vi "Magnetic Sweep 1.3.vi"() -> ()   [LabVIEW 2011]
uses:
  <vilib>/Math Plots/3D Math Plots/3D Contour/3D Contour XCtrl/3D Contour.xctl
  <vilib>/Math Plots/3D Math Plots/3D Contour/3D Contour Datatype/Public/Plot Helper (Vector).vi
  <vilib>/Math Plots/3D Math Plots/3D Contour/3D Contour Datatype/3D Contour Datatype.lvclass
panel:
  in  "Set parameter":bool
  out "status":string
  out "PID command":string
  out "setpoint command":string
  out "setpoint":dbl
  out "3D Contour \n(Ramp down)":refnum<class "3D Plot Datatype.lvclass">[](xcontrol)
  out "3D Contour\n(Ramp up)":refnum<class "3D Plot Datatype.lvclass">[](xcontrol)
  in  "stop":bool
  out "error out 3":errorcluster
  out "error out 2":errorcluster
  in  "Contour plot (ramp down)":path
  in  "Raw data (ramp down)":path
  out "Elapsed Time (s)":dbl
  out "Numeric":i32
  in  "error out":errorcluster
  out "Initial Temperature":string
  out "Zero field reached":bool
  out "Target field reached":bool
  in  "Upper limite":dbl
  in  "Temperature\nramping step":dbl
  in  "Heater range":i16(ring) items=["High", "Medium", "Low"]
  in  "D gain":dbl
  in  "I gain":dbl
  in  "P gain":dbl
  in  "Contour plot (ramp up)":path
  out "Time elapsed":string
  in  "Timer":bool caption="Reset"
  in  "date format":enum16{"short", "long", "abbreviated"}(ring)
  in  "Save":bool
  in  "Raw data (ramp  up)":path
  out "Temperature vs Time":cluster{dbl[], dbl[]}(graph)
  out "current time":timestamp
  out "Magnetic\nField":cluster{dbl[], dbl[]}(graph)
  out "Current Resistance":string
  out "Current Temperature":string
  out "Current Field":string
  out "Status":string
  in  "Field Sweep":bool
  in  "Magnetic field\nRamp rate":dbl
  in  "Traget Field":dbl
  out "Init Response":string
  in  "error in (no error)":errorcluster
  in  "IP Address":string
  in  "Ramp":bool
  in  "Update":bool
  in  "Ramp to Zero":bool
  in  "P Switch":bool
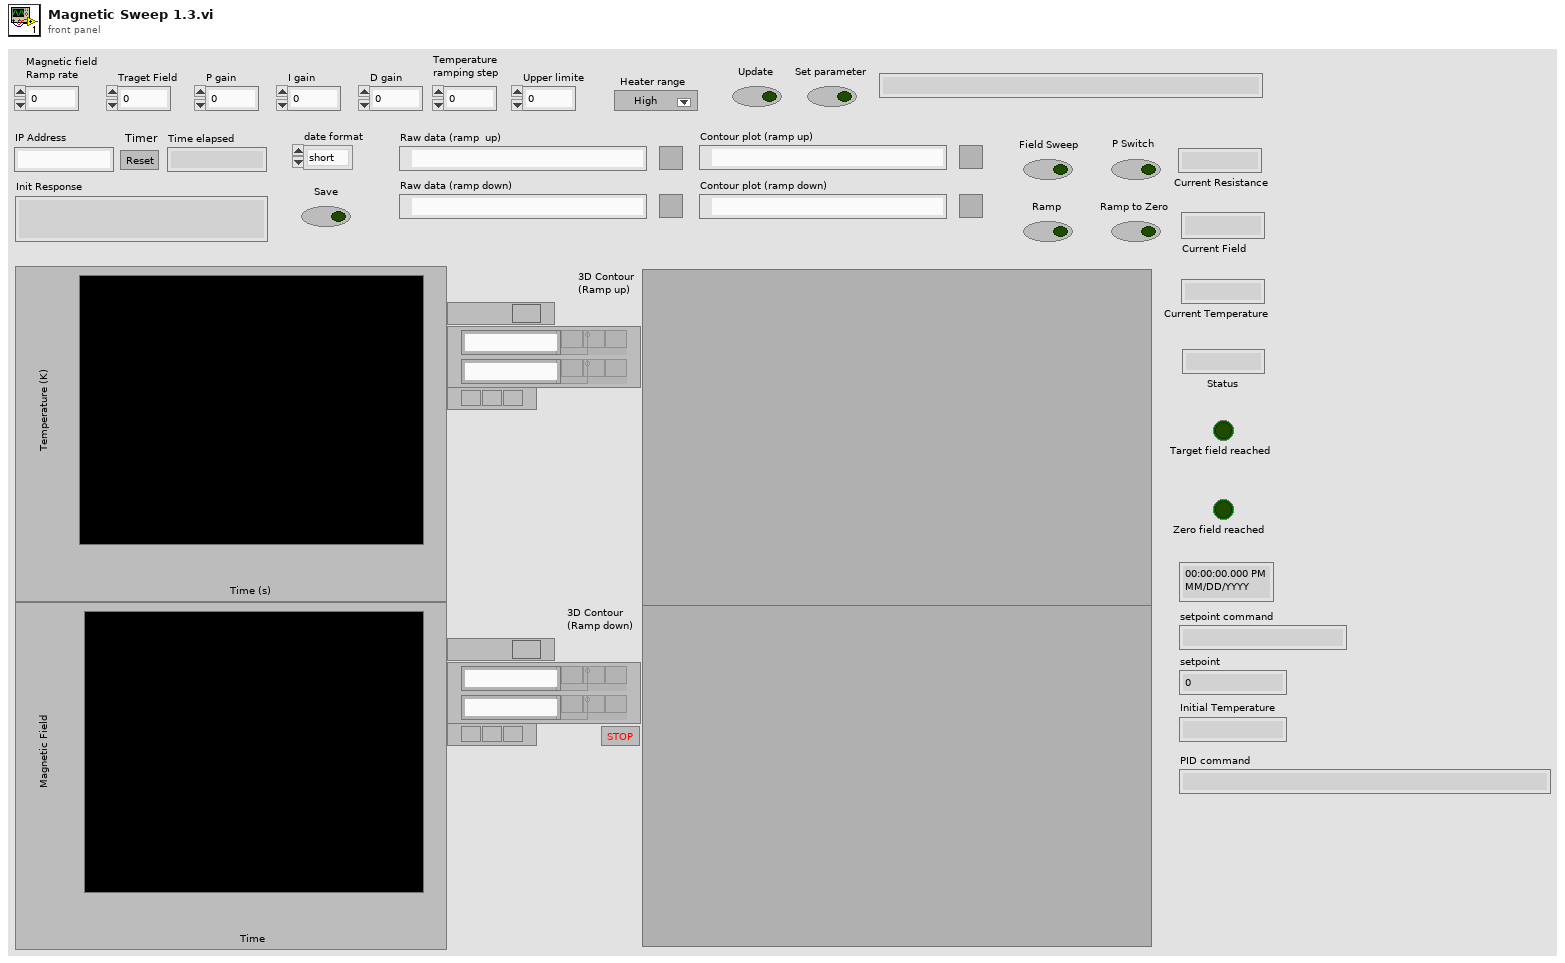
[diagram p1: front panel]
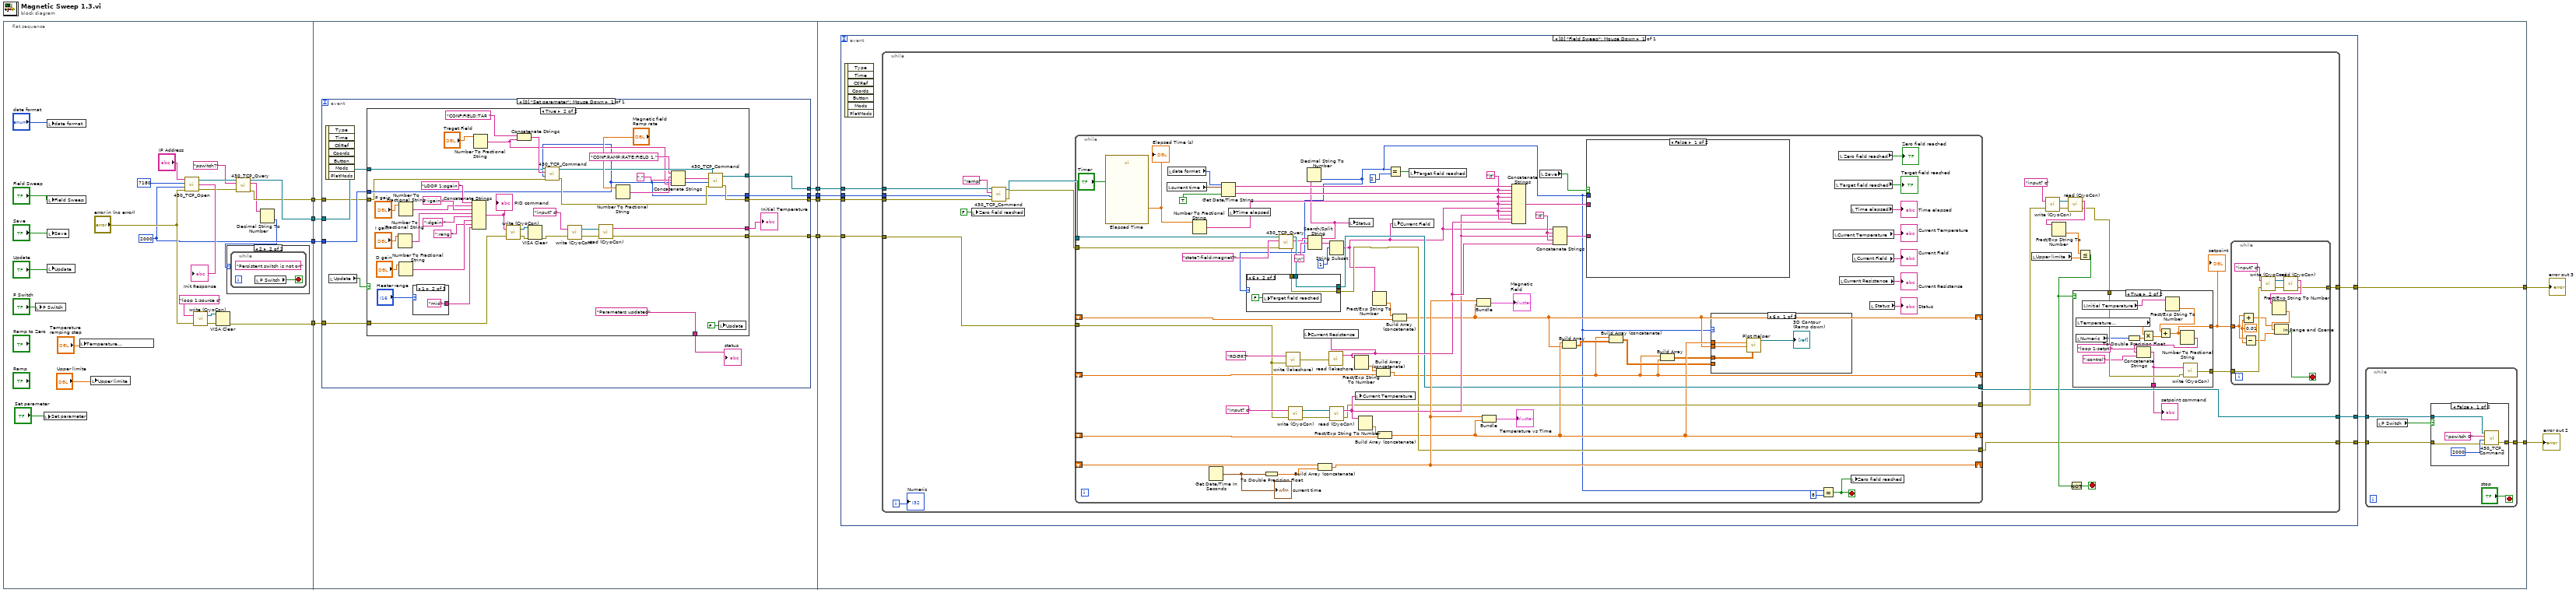
[diagram p0: block diagram]
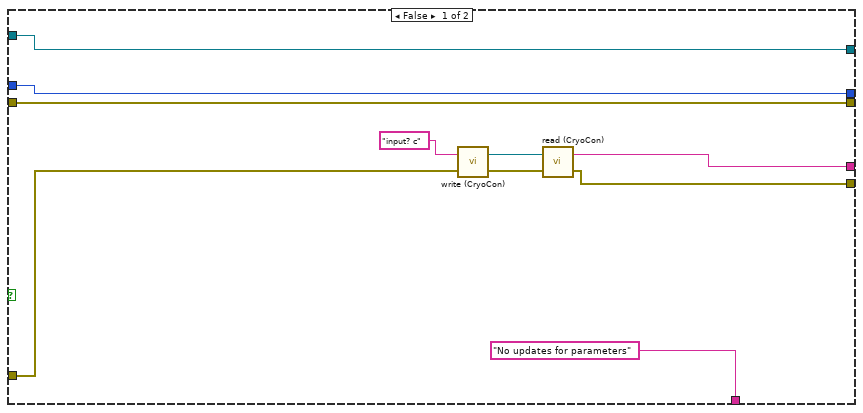
[diagram p3: hidden frame]
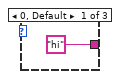
[diagram p4: hidden frame]
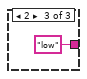
[diagram p5: hidden frame]
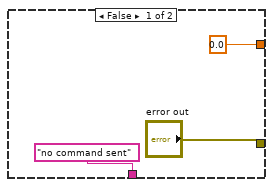
[diagram p7: hidden frame]
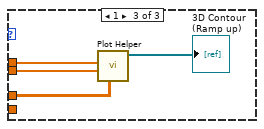
[diagram p9: hidden frame]
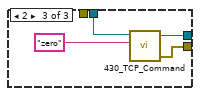
[diagram p11: hidden frame]
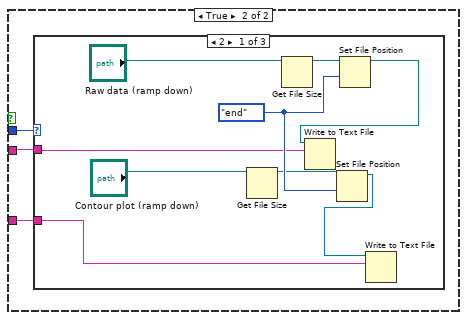
[diagram p12: hidden frame]
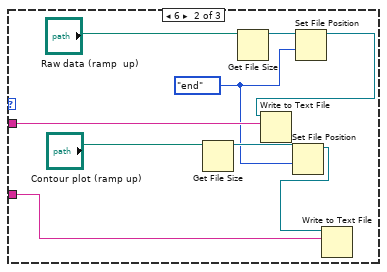
[diagram p13: hidden frame]
diagram:
  n1 = flat-sequence {
    tunnel: [w20] -> w10
    tunnel: [w22] -> w9
    tunnel: [w11] -> w8
    tunnel: [w18] -> w1
    tunnel: w10 -> [w43]
    tunnel: w9 -> [w42]
    tunnel: w8 -> [w41]
    tunnel: [w40] -> w7
    tunnel: [w39] -> w4
    tunnel: [w38] -> w3
    tunnel: [w37] -> w2
    tunnel: w1 -> [w36]
    tunnel: w7 -> [w115]
    tunnel: [w114] -> w6
    tunnel: [w112] -> w5
    tunnel: w4 -> [w110]
    tunnel: w3 -> [w109]
    tunnel: w2 -> [w108]
    frame #0 {
      w22 = 2000 ("Timeout")
      n2 = local write "P Switch"("P Switch") -> ()
      n3 = local write "Set parameter"("Set parameter") -> ()
      n4 = local write "date format"("date format") -> ()
      n5 = local write "Field Sweep"("Field Sweep") -> ()
      n6 = local write "Save"("Save") -> ()
      n7 = local write "Update"("Update") -> ()
      n8 = local write "Temperature\nramping step"("Temperature\nramping step") -> ()
      n9 = local write "Upper limite"("Upper limite") -> ()
      n10 = call "430_TCP_Open.vi"("IP Address"="IP Address", "TCP Port"=7180, "timeout ms (2000)"=w22, "error in (no error)"="error in (no error)") -> ("connection ID"=w21:refnum<k5>, "Init Response"=→"Init Response":string, "error out"=w19:errorcluster)  [unwired: 2 in]
      n11 = call "write (CryoCon).vi"("error in (no error)"="error in (no error)", "write buffer"="loop 1:source c") -> ("error out"=w13:errorcluster, "VISA resource name out"=w12:refnum<visa-resource-name>)
      n12 = VISA Clear(VISA resource name=w12, error in (no error)=w13) -> (error out=w11:errorcluster)  [unwired: 1 out]
      n13 = call "430_TCP_Query.vi"("error in (no error)"=w19, "Command"="pswitch?", "connection ID"=w21) -> ("error out"=w18:errorcluster, "Response"=w16:string, "connection ID out"=w20:refnum<k5>)  [unwired: 4 in, 2 out]
      n14 = Decimal String To Number(string=w16) -> (number=w15:i32)  [unwired: 2 in, 1 out]
      n15 = case shown="2" w15 {
        frame 1, Default {
        }
        frame 2 {
          n16 = while {
            stop <- w35 stop-if-true
            (unwired) "Persistent switch is not on"
            n17 = local read "P Switch"() -> (w35:bool)
          }
        }
      }
    }
    frame #1 {
      n18 = event shown="[0] \"Set parameter\": Mouse Down" {
        selector: _ -> [_]
        dyn-events: _ -> [_]
        timeout: _ -> [_]
        tunnel: w43 -> [w54]
        tunnel: w42 -> [w53]
        tunnel: w41 -> [w52]
        tunnel: [w51] -> w40
        tunnel: [w50] -> w39
        tunnel: [w49] -> w38
        tunnel: [w48] -> w37
        tunnel: w36 -> [w45]
        event "Set parameter": Mouse Down {
          n19 = event-data() -> ()  [unwired: 1 in, 7 out]
          n20 = local read "Update"() -> (w44:bool)
          n21 = case shown="True" w44 {
            tunnel: w54 -> [w62 w102]
            tunnel: w53 -> [w63 w72]
            tunnel: w52 -> [w56 w81]
            tunnel: [w61 w76] -> w51
            tunnel: ["No updates for parameters" ("String") "Parameters updated" ("String")] -> w47
            tunnel: [w55 w74] -> w50
            tunnel: [w62 w73] -> w49
            tunnel: [w63 w72] -> w48
            tunnel: [w58 w71] -> w46
            tunnel: w45 -> [w55 w68]
            frame False {
              n22 = call "write (CryoCon).vi"("error in (no error)"=w56, "write buffer"="input? c") -> ("error out"=w59:errorcluster, "VISA resource name out"=w57:refnum<visa-resource-name>)
              n23 = call "read (CryoCon).vi"("error in (no error)"=w59, "VISA resource name"=w57) -> ("error out"=w61:errorcluster, "read buffer"=w58:string)
            }
            frame True {
              n24 = Number To Fractional String(number="I gain") -> (F-format string=w85:string)  [unwired: 3 in]
              n25 = Number To Fractional String(number="D gain") -> (F-format string=w83:string)  [unwired: 3 in]
              n26 = Number To Fractional String(number="P gain") -> (F-format string=w86:string)  [unwired: 3 in]
              n27 = case shown="1" "Heater range" {
                tunnel: ["hi" "mid" "low"] -> w78
                frame 0, Default {
                }
                frame 1 {
                }
                frame 2 {
                }
              }
              n28 = Concatenate Strings("LOOP 1:pgain " ("write buffer"), w86, ";igain " ("string"), w85, ";dgain " ("string"), w83, ";rang " ("string"), w78) -> (w82:string)
              "PID command" <- w82
              n29 = Number To Fractional String(number="Traget Field") -> (F-format string=w92:string)  [unwired: 3 in]
              n30 = call "write (CryoCon).vi"("error in (no error)"=w81, "write buffer"=w82) -> ("error out"=w67:errorcluster, "VISA resource name out"=w66:refnum<visa-resource-name>)
              n31 = Concatenate Strings("CONF:FIELD:TAR ", w92) -> (w103:string)
              n32 = VISA Clear(VISA resource name=w66, error in (no error)=w67) -> (error out=w65:errorcluster)  [unwired: 1 out]
              n33 = call "430_TCP_Command.vi"("error in (no error)"=w68, "Timeout"=w72, "Command"=w103, "connection ID"=w102) -> ("error out"=w101:errorcluster, "connection ID out"=w97:refnum<k5>)  [unwired: 1 out]
              n34 = call "write (CryoCon).vi"("error in (no error)"=w65, "write buffer"="input? c") -> ("error out"=w77:errorcluster, "VISA resource name out"=w69:refnum<visa-resource-name>)
              n35 = call "read (CryoCon).vi"("error in (no error)"=w77, "VISA resource name"=w69) -> ("error out"=w76:errorcluster, "read buffer"=w71:string)
              n36 = Number To Fractional String(number="Magnetic field\nRamp rate") -> (F-format string=w95:string)  [unwired: 3 in]
              n37 = Concatenate Strings("CONF:RAMP:RATE:FIELD 1," ("string"), w95, "," ("string"), w92) -> (w98:string)
              n38 = call "430_TCP_Command.vi"("error in (no error)"=w101, "Timeout"=w72, "Command"=w98, "connection ID"=w97) -> ("error out"=w74:errorcluster, "connection ID out"=w73:refnum<k5>)  [unwired: 1 out]
              n39 = local write "Update"(FALSE ("Update")) -> ()
            }
          }
          "Initial Temperature" <- w46
          "status" <- w47
        }
      }
    }
    frame #2 {
      n40 = event shown="[0] \"Field Sweep\": Mouse Down" {
        selector: _ -> [_]
        dyn-events: _ -> [_]
        timeout: _ -> [_]
        tunnel: w115 -> [w133]
        tunnel: [w132] -> w114
        tunnel: [w131] -> w113
        tunnel: [w130] -> w111
        tunnel: w110 -> [w129]
        tunnel: w109 -> [w128]
        tunnel: w108 -> [w127]
        event "Field Sweep": Mouse Down {
          n41 = event-data() -> ()  [unwired: 1 in, 7 out]
          n42 = while {
            tunnel: w133 -> [w156]
            tunnel: [w140] -> w132
            tunnel: [w139] -> w131
            tunnel: [w138] -> w130
            tunnel: w129 -> [w136]
            tunnel: w128 -> [w135]
            tunnel: w127 -> [w134]
            i -> [w153]
            stop <- w142 stop-if-true
            n43 = local write "Zero field reached"(FALSE ("Zero field reached")) -> ()
            n44 = call "430_TCP_Command.vi"("error in (no error)"=w136, "Timeout"=w134, "Command"="ramp", "connection ID"=w135) -> ("error out"=w158:errorcluster, "connection ID out"=w157:refnum<k5>)  [unwired: 1 out]
            n45 = while {
              shift-right: [w192] -> _
              shift-left: _ -> [w242]
              shift-right: [w193] -> _
              shift-left: _ -> [w247]
              shift-right: [w189] -> _
              shift-left: _ -> [w244]
              shift-right: [w237] -> _
              shift-left: _ -> [w238]
              tunnel: w158 -> [w226]
              tunnel: w157 -> [w225]
              tunnel: w156 -> [w219]
              tunnel: [w213] -> w143
              tunnel: [w202] -> w139
              tunnel: [w201] -> w138
              stop <- w205 stop-if-true
              w230 = "\t"
              w231 = "\t"
              n46 = call "Elapsed Time"("Reset"="Timer") -> ("Elapsed Time (s)"=w217:dbl)  [unwired: 11 in, 7 out]
              "Elapsed Time (s)" <- w217
              n47 = local read "current time"() -> (w228:timestamp)
              n48 = local read "date format"() -> (w220:enum16{"short", "long", "abbreviated"})
              n49 = Number To Fractional String(number=w217) -> (F-format string=w223:string)  [unwired: 3 in]
              n50 = Get Date/Time In Seconds() -> (seconds since 1Jan1904=w216:timestamp)
              "current time" <- w216
              n51 = Get Date/Time String(date format (0)=w220, seconds (now)=w228, want seconds? (F)=TRUE) -> (date string=w233:string, time string=w232:string)
              n52 = local write "Time elapsed"(w223) -> ()
              n53 = To Double Precision Float(number=w216) -> (double precision float=w239:dbl)
              n54 = call "430_TCP_Query.vi"("error in (no error)"=w226, "Command"="state?;field:magnet?", "connection ID"=w225) -> ("error out"=w187:errorcluster, "Response"=w200:string, "connection ID out"=w204:refnum<k5>)  [unwired: 4 in, 2 out]
              n55 = call "write (lakeshore).vi"("error in (no error)"=w219, "write buffer"="RDGR?") -> ("error out"=w246:errorcluster)
              n56 = call "write (CryoCon).vi"("error in (no error)"=w219, "write buffer"="input? c") -> ("error out"=w248:errorcluster, "VISA resource name out"=w249:refnum<visa-resource-name>)
              n57 = Search/Split String(string=w200, search string/char (-)="\n") -> (substring before match=w199:string, match + rest of string=w198:string)  [unwired: 1 in, 1 out]
              n58 = Decimal String To Number(string=w199) -> (number=w188:i32)  [unwired: 2 in, 1 out]
              n59 = case shown="6" w188 {
                tunnel: [w260 w262 w267] -> w201
                tunnel: w204 -> [w261 w264 w266]
                tunnel: [w261 w264 w265] -> w202
                tunnel: w187 -> [w260 w262 _]
                frame 0, Default {
                }
                frame 6 {
                  n60 = local write "Target field reached"(FALSE ("Target field reached")) -> ()
                }
                frame 2 {
                  n61 = call "430_TCP_Command.vi"("Command"="zero", "connection ID"=w266) -> ("error out"=w267:errorcluster, "connection ID out"=w265:refnum<k5>)  [unwired: 2 in, 1 out]
                }
              }
              n62 = Build Array (concatenate)(w238, w239) -> (w237:dbl[])
              n63 = call "read (lakeshore).vi"("error in (no error)"=w246) -> ("read buffer"=w222:string)  [unwired: 1 out]
              n64 = local write "Current Resistance"(w222) -> ()
              n65 = String Subset(string=w198, offset (0)=1) -> (substring=w196:string)  [unwired: 1 in]
              n66 = call "read (CryoCon).vi"("error in (no error)"=w248, "VISA resource name"=w249) -> ("error out"=w213:errorcluster, "read buffer"=w221:string)
              n67 = local write "Status"(w199) -> ()
              n68 = Fract/Exp String To Number(string=w222) -> (number=w240:dbl)  [unwired: 3 in, 1 out]
              n69 = local write "Current Temperature"(w221) -> ()
              n70 = Fract/Exp String To Number(string=w221) -> (number=w241:dbl)  [unwired: 3 in, 1 out]
              n71 = Fract/Exp String To Number(string=w196) -> (number=w243:dbl)  [unwired: 3 in, 1 out]
              n72 = Build Array (concatenate)(w240, w244) -> (w189:dbl[])
              n73 = Build Array (concatenate)(w241, w247) -> (w193:dbl[])
              n74 = Equal?(x=w188, y=2) -> (x = y?=w224:bool)
              n75 = Build Array (concatenate)(w243, w242) -> (w192:dbl[])
              n76 = local write "Current Field"(w196) -> ()
              n77 = local write "Target field reached"(w224) -> ()
              n78 = Bundle(w237, w192) -> (→"Magnetic\nField":cluster{dbl[], dbl[]})  [unwired: 1 in]
              n79 = Bundle(w237, w193) -> (→"Temperature vs Time":cluster{dbl[], dbl[]})  [unwired: 1 in]
              n80 = Concatenate Strings(w233, w231, w232, w231, w223, w231, w196, w231, w221, w231, w222) -> (w236:string)
              n81 = local read "Save"() -> (w215:bool)
              n82 = Concatenate Strings(w196, w230, w221, w230, w222) -> (w229:string)
              n83 = Build Array(w193, w192) -> (w203:dbl[][])
              n84 = case shown="False" w215 {
                tunnel: w236 -> [_ w271]
                tunnel: w229 -> [_ w270]
                tunnel: w188 -> [_ w269]
                frame False {
                }
                frame True {
                  n85 = case shown="2" w269 {
                    tunnel: w271 -> [w273 w289 _]
                    tunnel: w270 -> [w272 w283 _]
                    frame 2 {
                      w279 = enum16{"start", "end", "current"}."end" ("from (0:start)")
                      n86 = Get File Size(file="Contour plot (ramp down)") -> (refnum out=w278:refnum<file>)  [unwired: 1 in, 2 out]
                      n87 = Get File Size(file="Raw data (ramp down)") -> (refnum out=w275:refnum<file>)  [unwired: 1 in, 2 out]
                      n88 = Set File Position(refnum=w278, from (0:start)=w279) -> (refnum out=w280:refnum<file>)  [unwired: 2 in, 1 out]
                      n89 = Set File Position(refnum=w275, from (0:start)=w279) -> (refnum out=w276:refnum<file>)  [unwired: 2 in, 1 out]
                      n90 = Write to Text File(file (use dialog)=w276, text=w273) -> ()  [unwired: 2 in, 3 out]
                      n91 = Write to Text File(file (use dialog)=w280, text=w272) -> ()  [unwired: 2 in, 3 out]
                    }
                    frame 6 {
                      w282 = enum16{"start", "end", "current"}."end" ("from (0:start)")
                      n92 = Get File Size(file="Contour plot (ramp up)") -> (refnum out=w284:refnum<file>)  [unwired: 1 in, 2 out]
                      n93 = Get File Size(file="Raw data (ramp  up)") -> (refnum out=w287:refnum<file>)  [unwired: 1 in, 2 out]
                      n94 = Set File Position(refnum=w284, from (0:start)=w282) -> (refnum out=w281:refnum<file>)  [unwired: 2 in, 1 out]
                      n95 = Set File Position(refnum=w287, from (0:start)=w282) -> (refnum out=w286:refnum<file>)  [unwired: 2 in, 1 out]
                      n96 = Write to Text File(file (use dialog)=w286, text=w289) -> ()  [unwired: 2 in, 3 out]
                      n97 = Write to Text File(file (use dialog)=w281, text=w283) -> ()  [unwired: 2 in, 3 out]
                    }
                    frame Default {
                    }
                  }
                }
              }
              n98 = Build Array (concatenate)(w189, w203) -> (w190:dbl[][])
              n99 = Build Array(w189, w189) -> (w191:dbl[][])
              n100 = case shown="6" w188 {
                tunnel: w193 -> [w254 _ w258]
                tunnel: w192 -> [w253 _ w257]
                tunnel: w191 -> [w252 _ w256]
                tunnel: w190 -> [_ _ _]
                frame 6 {
                  n101 = call-poly <vilib>:"Plot Helper.vi"("z matrix"=w252, "y vector"=w253, "x vector"=w254) -> ("3D Plot lvclass Array out"=→"3D Contour \n(Ramp down)":refnum<class "3D Plot Datatype.lvclass">[])  [unwired: 3 in, 5 out]
                }
                frame 0, Default {
                }
                frame 1 {
                  n102 = call-poly <vilib>:"Plot Helper.vi"("z matrix"=w256, "y vector"=w257, "x vector"=w258) -> ("3D Plot lvclass Array out"=→"3D Contour\n(Ramp up)":refnum<class "3D Plot Datatype.lvclass">[])  [unwired: 3 in, 5 out]
                }
              }
              n103 = Equal?(x=w188, y=8) -> (x = y?=w205:bool)
              n104 = local read "Current Temperature"() -> (→"Current Temperature":string)
              n105 = local read "Target field reached"() -> (→"Target field reached":bool)
              n106 = local read "Zero field reached"() -> (→"Zero field reached":bool)
              n107 = local read "Current Resistance"() -> (→"Current Resistance":string)
              n108 = local read "Time elapsed"() -> (→"Time elapsed":string)
              n109 = local write "Zero field reached"(w205) -> ()
              n110 = local read "Current Field"() -> (→"Current Field":string)
              n111 = local read "Status"() -> (→"Status":string)
            }
            n112 = local read "Upper limite"() -> (w145:dbl)
            n113 = call "write (CryoCon).vi"("error in (no error)"=w143, "write buffer"="input? c") -> ("error out"=w148:errorcluster, "VISA resource name out"=w149:refnum<visa-resource-name>)
            n114 = call "read (CryoCon).vi"("error in (no error)"=w148, "VISA resource name"=w149) -> ("error out"=w146:errorcluster, "read buffer"=w147:string)
            n115 = Fract/Exp String To Number(string=w147) -> (number=w144:dbl)  [unwired: 3 in, 1 out]
            n116 = Less Or Equal?(x=w144, y=w145) -> (x <= y?=w141:bool)
            n117 = Not(x=w141) -> (.not. x?=w142:bool)
            n118 = case shown="True" w141 {
              tunnel: w146 -> [_ w184]
              tunnel: ["error out" w181] -> w155
              tunnel: [0.0 w180] -> w154
              tunnel: ["no command sent" w174] -> w137
              frame False {
              }
              frame True {
                n119 = local read "Temperature\nramping step"() -> (w178:dbl)
                n120 = local read "Numeric"() -> (w176:i32)
                n121 = local read "Initial Temperature"() -> (w183:string)
                n122 = To Double Precision Float(number=w176) -> (double precision float=w177:dbl)
                n123 = Multiply(x=w178, y=w177) -> (x*y=w179:dbl)
                n124 = Fract/Exp String To Number(string=w183) -> (number=w182:dbl)  [unwired: 3 in, 1 out]
                n125 = Add(x=w182, y=w179) -> (x+y=w180:dbl)
                n126 = Number To Fractional String(number=w180) -> (F-format string=w185:string)  [unwired: 3 in]
                n127 = Concatenate Strings("loop 1:setpt " ("write buffer"), w185, ";control" ("string")) -> (w174:string)
                n128 = call "write (CryoCon).vi"("error in (no error)"=w184, "write buffer"=w174) -> ("error out"=w181:errorcluster)  [unwired: 1 out]
              }
            }
            "setpoint" <- w154
            "setpoint command" <- w137
            n129 = while {
              tunnel: w155 -> [w169]
              tunnel: w154 -> [w164]
              tunnel: [w159] -> w140
              stop <- w160 stop-if-true
              w161 = 0.01 ("y")
              n130 = Add(x=w164, y=w161) -> (x+y=w163:dbl)
              n131 = Subtract(x=w164, y=w161) -> (x-y=w162:dbl)
              n132 = call "write (CryoCon).vi"("error in (no error)"=w169, "write buffer"="input? c") -> ("error out"=w168:errorcluster, "VISA resource name out"=w170:refnum<visa-resource-name>)
              n133 = call "read (CryoCon).vi"("error in (no error)"=w168, "VISA resource name"=w170) -> ("error out"=w159:errorcluster, "read buffer"=w166:string)
              n134 = Fract/Exp String To Number(string=w166) -> (number=w165:dbl)  [unwired: 3 in, 1 out]
              n135 = In Range and Coerce(upper limit=w163, x=w165, lower limit=w162) -> (In Range?=w160:bool)  [unwired: 1 out]
            }
            "Numeric" <- w153
          }
        }
      }
      n136 = while {
        tunnel: w113 -> [w120]
        tunnel: [w118] -> w112
        tunnel: w111 -> [w117]
        stop <- "stop" stop-if-true
        n137 = local read "P Switch"() -> (w119:bool)
        n138 = case shown="False" w119 {
          tunnel: w120 -> [w124 _]
          tunnel: [w122 w126] -> w118
          tunnel: w117 -> [w121 w126]
          frame False {
            n139 = call "430_TCP_Command.vi"("error in (no error)"=w121, "Timeout"=2000, "Command"="pswitch 0", "connection ID"=w124) -> ("error out"=w122:errorcluster)  [unwired: 2 out]
          }
          frame True {
          }
        }
      }
    }
  }
  "error out 2" <- w5
  "error out 3" <- w6
